vi "Copy Image to Memory Address.vi"   [LabVIEW 2020, in "g_ar_toolkit.image.lvlib"]
doc: "Copy a LabVIEW Pixmap Image to an ARGB or Greyscale image with the option to generate a mask from the mask data in the Pixmap.\n\nOnly 8, 24 and 32-bit image depths are supported."
uses:
  g_ar_toolkit.image.lvlib
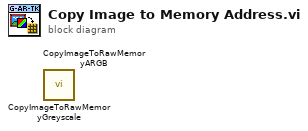
[diagram p0: block diagram]
diagram:
  n1 = call "CopyImageToRawMemoryGreyscale.vi"() -> ()  [unwired: 10 in, 2 out]
  n2 = call "CopyImageToRawMemoryARGB.vi"() -> ()  [unwired: 10 in, 2 out]
